vi "All Created Events.vi"(9 "Priority?":bool, 10 "Msg Strategy":refnum<class "Msg Strategy.lvclass">, 11 "Base Queue in":refnum<class "Base Queue.lvclass">) -> (3 "Base Queue out":refnum<class "Base Queue.lvclass">)   [LabVIEW 2021, in "jettl.lvlib" / "Base Queue.lvlib" / "Base Queue.lvclass"]
uses:
  Base Queue.lvclass
  Msg Strategy/Msg Strategy.lvclass
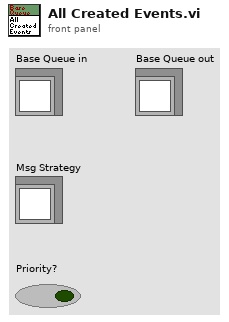
[diagram p1: front panel]
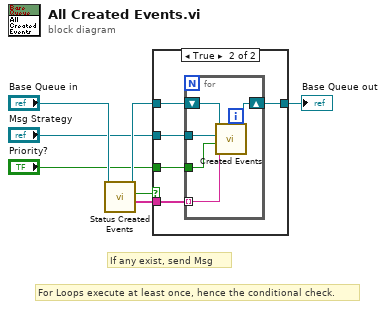
[diagram p0: block diagram]
diagram:
  # "If any exist, send Msg"
  # "For Loops execute at least once, hence the conditional check."
  n1 = call-dynamic "Status Created Events.vi"("Base Queue in"="Base Queue in") -> ("Created Event Aliases"=w4:string[], "Created Event Exist?"=w5:bool, "Base Queue out"=w3:refnum<class "Base Queue.lvclass">)  [unwired: 7 in, 1 out]
  n2 = case shown="True" w5 {
    tunnel: [w8 w13] -> w7
    tunnel: w3 -> [w8 w12]
    tunnel: w4 -> [_ w11]
    tunnel: "Msg Strategy" -> [_ w10]
    tunnel: "Priority?" -> [_ w9]
    frame False {
    }
    frame True {
      n3 = for {
        tunnel: w11 -> [w16] mode=indexing
        shift-right: [w18] -> w13
        shift-left: w12 -> [w17]
        tunnel: w10 -> [w15]
        tunnel: w9 -> [w14]
        n4 = call-dynamic "Created Events.vi"("Created Event Alias"=w16, "Priority?"=w14, "Msg Strategy"=w15, "Base Queue in"=w17) -> ("Base Queue out"=w18:refnum<class "Base Queue.lvclass">)  [unwired: 7 in]
      }
    }
  }
  "Base Queue out" <- w7
